vi "SetDualPass.vi"(0 "Dual Pass Cluster":T1={"Alternative Setpoint"=-2147483648, "Setpoint"=-inf, "Alternative DAC"=-2147483648, "Number of DAC"=3, "Value of DAC"=-2147483648, "Alternative Fexc"=-2147483648, "Value of Fexc"=-inf, "Lift Offset"=-inf, "Wait Time"=-inf, "Lift Slewrate"=-inf} {"Lift Slewrate" format="%#_g V/s"; "Wait Time" format="%#_g ms"; "Lift Offset" format="%#_g nm"; "Value of Fexc" format="%#_g kHz"; "Alternative Fexc" items=["[read only]"=-2147483648, "No"=0, "Yes"=1]; "Value of DAC" format="%.0f V"; "Number of DAC" items=["DAC 1", "DAC 2", "DAC 3", "DAC 4"]; "Alternative DAC" items=["[read only]"=-2147483648, "No"=0, "Yes"=1]; "Alternative Setpoint" items=["[read only]"=-2147483648, "No"=0, "Yes"=1]}, 5 "error in":T6) -> (14 "Output Cluster":T1={"Alternative Setpoint"=-2147483648, "Setpoint"=-inf, "Alternative DAC"=-2147483648, "Number of DAC"=0, "Value of DAC"=-2147483648, "Alternative Fexc"=-2147483648, "Value of Fexc"=-inf, "Lift Offset"=-inf, "Wait Time"=-inf, "Lift Slewrate"=-inf} {"Lift Slewrate" format="%#_g V/s"; "Wait Time" format="%#_g ms"; "Lift Offset" format="%#_g nm"; "Value of Fexc" format="%#_g kHz"; "Alternative Fexc" items=["[read only]"=-2147483648, "No"=0, "Yes"=1]; "Value of DAC" format="%.0f V"; "Number of DAC" items=["DAC 1", "DAC 2", "DAC 3", "DAC 4"]; "Alternative DAC" items=["[read only]"=-2147483648, "No"=0, "Yes"=1]; "Alternative Setpoint" items=["[read only]"=-2147483648, "No"=0, "Yes"=1]}, 19 "error out":T6)   [LabVIEW 2016]
doc: "Sets the parameters for the second pass mode. The 'Dual Pass Cluster' contains the following values:\n- Alternative Setpoint (integer) [0 -- no; 1 -- yes]\n- Setpoint (float) [without restraint]\n- Alternative DAC (integer) [0 -- no; 1 --yes]\n- Number of DAC (integer) [0-3 -- DAC1-4] required input\n- Value of DAC in V(float) [-10 to 10]\n- Alternative Fexc (integer) [0 -- no; 1 --yes]\n- Value of Fexc (float) [0 to 2000]\n- Lift Offset (float) [0 to 1000000]\n- Wait Time (float) [without restraint]\n- Lift Slewrate (float) [0.001863 to 1000]\n\nThe 'Alternative Setpoint' flag activates or deactivates the use of an alternative setpoint. Its value would be given by 'setpoint'. The same applies for the fexc and an alternative DAC, with the constraint for the DAC that the number of it has to be specified as 'Number of DAC'. The output \"input = output\" indicates if in- and output-cluster contain the same values. If this is not the case at least one of the entered values has not been accepted by the server. By passing -Inf (float) or -2147483648 (integer) as input values, the corresponding parameter(s) will be read out."
uses:
  Controls/Dual-Pass_Parameters.ctl
  Controls/Dual-Pass-Alternative-Setpoint_Selection.ctl
  Controls/Dual-Pass-Alternative-DAC_Selection.ctl
  Controls/DAC_Selection.ctl
  Controls/Dual-Pass-Alternative-Fexc_Selection.ctl
  Controls/Error_Out.ctl
  Files_ASC500/DLL/ASC500_RemoteControlV27.dll
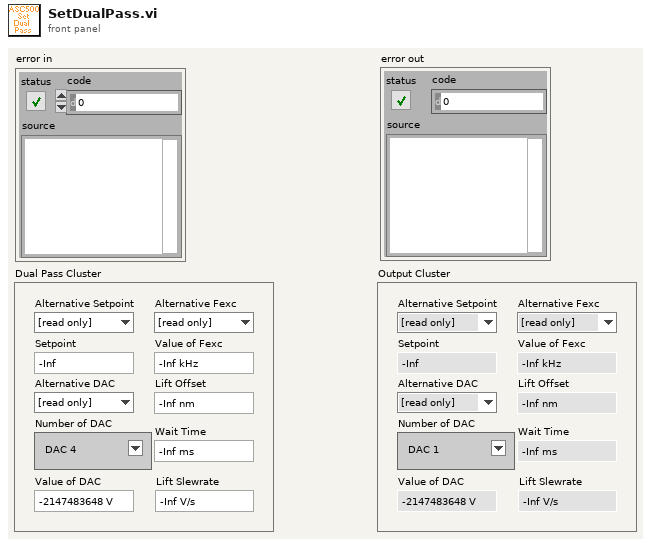
[diagram p1: front panel]
types:
  T1 = typedef "Dual-Pass_Parameters.ctl" = cluster{"Alternative Setpoint":T2, "Setpoint":sgl, "Alternative DAC":T3, "Number of DAC":T4, "Value of DAC":i32, "Alternative Fexc":T5, "Value of Fexc":sgl, "Lift Offset":sgl, "Wait Time":sgl, "Lift Slewrate":sgl}
  T2 = typedef "Dual-Pass-Alternative-Setpoint_Selection.ctl" = i32
  T3 = typedef "Dual-Pass-Alternative-DAC_Selection.ctl" = i32
  T4 = typedef "DAC_Selection.ctl" = u16
  T5 = typedef "Dual-Pass-Alternative-Fexc_Selection.ctl" = i32
  T6 = typedef "Error_Out.ctl" = errorcluster
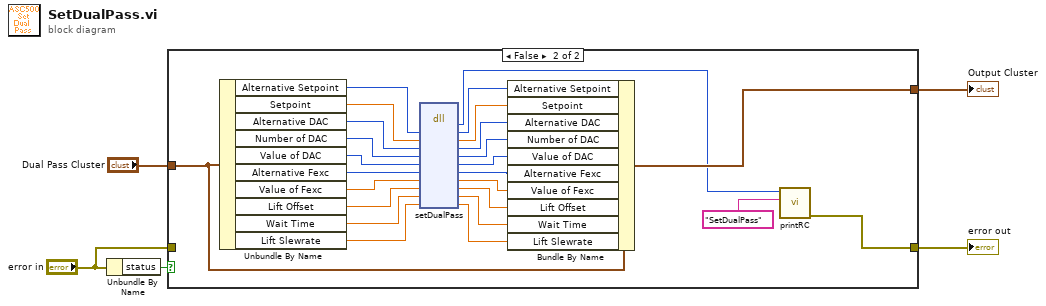
[diagram p0: block diagram]
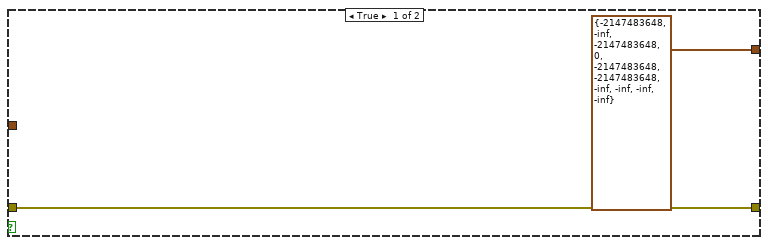
[diagram p2: hidden frame]
diagram:
  n1 = Unbundle By Name("error in") -> ("status"=w5:bool)
  n2 = case shown="False" w5 {
    tunnel: [w6 w10] -> w4
    tunnel: "Dual Pass Cluster" -> [_ w13]
    tunnel: [T1 {"Alternative Setpoint"=-2147483648, "Setpoint"=-inf, "Alternative DAC"=-2147483648, "Number of DAC"=0, "Value of DAC"=-2147483648, "Alternative Fexc"=-2147483648, "Value of Fexc"=-inf, "Lift Offset"=-inf, "Wait Time"=-inf, "Lift Slewrate"=-inf} ("Dual Pass Cluster") w12] -> w1
    tunnel: "error in" -> [w6 _]
    frame True {
    }
    frame False {
      n3 = Unbundle By Name(w13) -> ("Alternative Setpoint"=w32:T2, "Setpoint"=w31:sgl, "Alternative DAC"=w30:T3, "Number of DAC"=w29:T4, "Value of DAC"=w28:i32, "Alternative Fexc"=w27:T5, "Value of Fexc"=w26:sgl, "Lift Offset"=w25:sgl, "Wait Time"=w11:sgl, "Lift Slewrate"=w24:sgl)
      n4 = dll-call lib="G:/SCMOperations/Share/ELE/Produkt Information/ASC500/04 Remote Control/02 development versions/2018Nov06/Files_ASC500/DLL/ASC500_RemoteControlV27.dll" fn="setDualPass"("Alternative Setpoint"=w32, "Setpoint"=w31, "Alternative DAC"=w30, "Number of DAC"=w29, "Value of DAC"=w28, "Alternative Fexc"=w27, "Value of Fexc"=w26, "Lift Offset"=w25, "Wait Time"=w11, "Lift Slewrate"=w24) -> ("return type"=w9:i32, "Alternative Setpoint"=w23:i32, "Setpoint"=w22:sgl, "Alternative DAC"=w21:i32, "Number of DAC"=w20:i32, "Value of DAC"=w19:i32, "Alternative Fexc"=w18:i32, "Value of Fexc"=w17:sgl, "Lift Offset"=w16:sgl, "Wait Time"=w15:sgl, "Lift Slewrate"=w14:sgl)  [unwired: 3 in, 2 out]
      n5 = Bundle By Name(cluster=w13, "Alternative Setpoint"=w23, "Setpoint"=w22, "Alternative DAC"=w21, "Number of DAC"=w20, "Value of DAC"=w19, "Alternative Fexc"=w18, "Value of Fexc"=w17, "Lift Offset"=w16, "Wait Time"=w15, "Lift Slewrate"=w14) -> (w12:T1)
      n6 = call "printRC.vi"("additional information"="SetDualPass", "RC"=w9) -> ("error out"=w10:T6)  [unwired: 9 in]
    }
  }
  "error out" <- w4
  "Output Cluster" <- w1
